vi "PAS_CmdStr_191.vi"(1 "PAS动作输入":T1 {"APA泊车进度" max=100.0 step=2.0 scale=0.0..100.0; "自动泊车状态" items=["关闭", "待机", "搜索", "引导搜索", "完成", "失败", "终止", "无效"]; "指示泊车辅助被激活功能" items=["无激活", "pPSC激活", "cPSC激活", "POC激活", "预留"]; "指示当前选中的位置" items=["无", "左", "右", "预留"]; "SVA辅视系统工作模式" items=["关闭", "待机", "激活", "失败", "抑制", "预留"]; "停车位查找状况" items=["No Slot", "Slot_Left", "Slot_Right", "Invalid"]; "驱动请求状态" items=["No Request", "Req_Forward_Again", "Req_Turn_lever", "Req_Gear_P", "Req_Confirm_Switch", "Req_SearchingProcess", "Req_Drive_Fw", "Req_Stop", "Req_PEB", "Reserved", "Req_Function Select", "Req_Function off", "Req_Process bar", "pPSC request only", "cPSC request only", "pPSC&cPSC request", "Req_Gear_R", "Req_Gear_D", "Req_Drive_Bw", "Req_Slow_Down", "Req_Release Brake", "Req_Close Door", "Req_Buckle Seat Belt", "Req_Repress Dead Man Switch", "Req_Press Brake Pedal", "Req_Gear R and Brake"]; "APA可恢复中断退出提示" items=["No Request", "Req_Recover_Dead Man Switch Release", "Reserved", "Req_Recover_Non-Driver-Door Open", "Req_Recover_Found Obstacle In Trajectory", "Req_Recover_Steering Wheel Hands-On"]; "APA完全退出提示" items=["No Request", "Req_Quit_External ECU Failure", "Req_Quit_PAS_Failure", "Req_Quit_Speed high", "Req_Quit_Timing overflow", "Req_Quit_Move times overflow", "Req_Quit_Recover_Int_Tims_Overflow", "Req_Quit_Gas pedal", "Req_Quit_Gear Intervention", "Req_Quit_External ECU active", "Req_Quit_ACC", "Req_Quit_Trajectory", "Reserved", "Req_Quit_Space limit", "Req_Quit_No object in front", "Req_Quit_Seat belt unbunckle", "Req_Quit_Driver_Door", "Req_Quit_EPB_Apply", "Req_Quit_Vehicle Block", "Req_Quit_Gear Interrupt"]}) -> (0 "CmdStr":string)   [LabVIEW 2013]
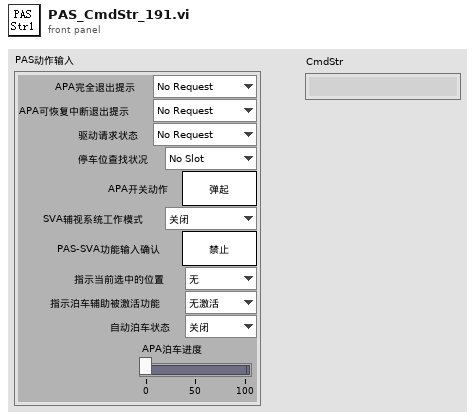
[diagram p1: front panel]
types:
  T1 = cluster{"APA完全退出提示":u8, "APA可恢复中断退出提示":u8, "驱动请求状态":u8, "停车位查找状况":u8, "APA开关动作":bool, "SVA辅视系统工作模式":u8, "PAS-SVA功能输入确认":bool, "指示当前选中的位置":u8, "指示泊车辅助被激活功能":u8, "自动泊车状态":u8, "APA泊车进度":dbl}
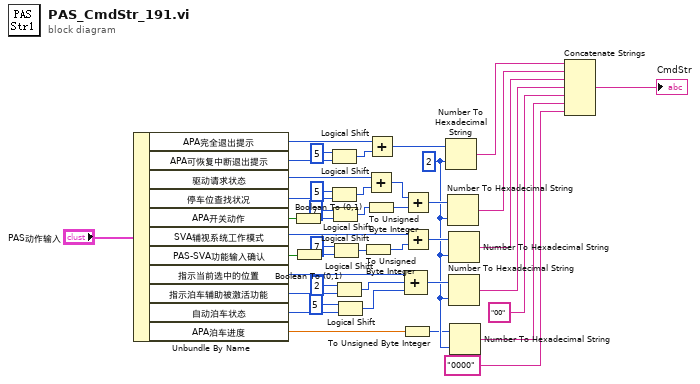
[diagram p0: block diagram]
diagram:
  w7 = 2
  n1 = Unbundle By Name("PAS动作输入") -> ("APA完全退出提示"=w42:u8, "APA可恢复中断退出提示"=w40:u8, "驱动请求状态"=w36:u8, "停车位查找状况"=w38:u8, "APA开关动作"=w34:bool, "SVA辅视系统工作模式"=w24:u8, "PAS-SVA功能输入确认"=w27:bool, "指示当前选中的位置"=w22:u8, "指示泊车辅助被激活功能"=w19:u8, "自动泊车状态"=w16:u8, "APA泊车进度"=w3:dbl)
  n2 = Boolean To (0,1)(Boolean=w34) -> (0, 1=w33:i16)
  n3 = Boolean To (0,1)(Boolean=w27) -> (0, 1=w28:i16)
  n4 = Logical Shift(y=u8 5, x=w40) -> (x << y=w41:u8)
  n5 = Logical Shift(y=u8 5, x=w38) -> (x << y=w35:u8)
  n6 = Logical Shift(y=u8 7, x=w33) -> (x << y=w30:i16)
  n7 = Logical Shift(y=u8 7, x=w28) -> (x << y=w26:i16)
  n8 = Logical Shift(y=u8 2, x=w19) -> (x << y=w21:u8)
  n9 = Logical Shift(y=u8 5, x=w16) -> (x << y=w20:u8)
  n10 = To Unsigned Byte Integer(number=w26) -> (unsigned 8bit integer=w25:u8)
  n11 = Add(x=w36, y=w35) -> (x+y=w31:u8)
  n12 = To Unsigned Byte Integer(number=w30) -> (unsigned 8bit integer=w29:u8)
  n13 = Add(x=w42, y=w41) -> (x+y=w14:u8)
  n14 = To Unsigned Byte Integer(number=w3) -> (unsigned 8bit integer=w4:u8)
  n15 = Add(x=w31, y=w29) -> (x+y=w12:u8)
  n16 = Add(x=w24, y=w25) -> (x+y=w11:u8)
  n17 = Compound Arithmetic op=ADD(w22, w21, w20) -> (w9:u8)
  n18 = Number To Hexadecimal String(1:w7, 2:w14) -> (0:w13:string)
  n19 = Number To Hexadecimal String(1:w7, 2:w12) -> (0:w15:string)
  n20 = Number To Hexadecimal String(1:w7, 2:w11) -> (0:w10:string)
  n21 = Number To Hexadecimal String(1:w7, 2:w9) -> (0:w8:string)
  n22 = Number To Hexadecimal String(1:w7, 2:w4) -> (0:w6:string)
  n23 = Concatenate Strings(w13, w15, w10, w8, "00", w6, "0000") -> (→"CmdStr":string)
